vi "JSON File Parse String.vi"(8 "error in (no error)":errorcluster, 11 "file json string":string) -> (0 "error out":errorcluster, 1 "version substring":string, 2 "dsf version substring":string, 3 "dsf configuration substring":string)   [LabVIEW 2017, in "DSF Core.lvlib" / "Configuration Session.lvclass"]
uses:
  Configuration Session.lvclass
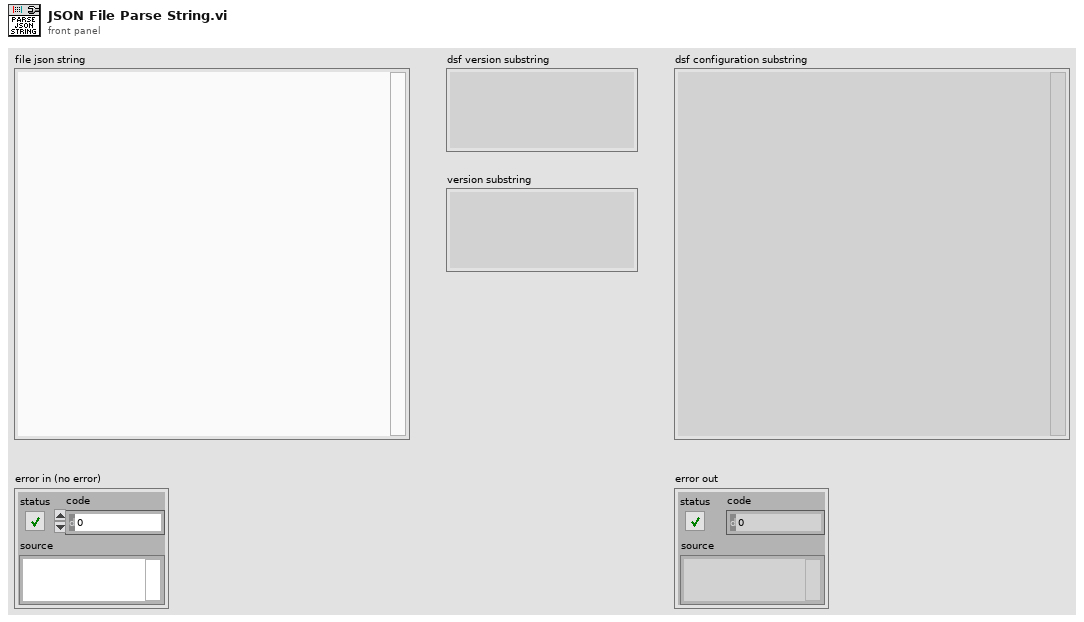
[diagram p1: front panel]
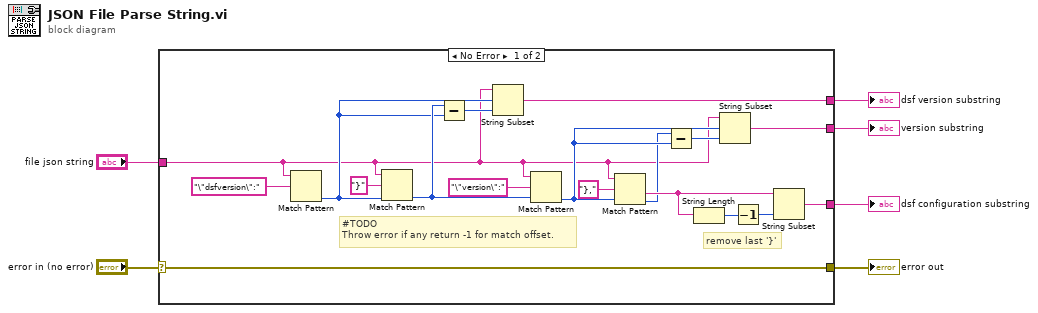
[diagram p0: block diagram]
diagram:
  n1 = case shown="No Error" "error in (no error)" {
    selector: "error in (no error)" -> [w10 w25]
    tunnel: [w19 _] -> w6
    tunnel: "file json string" -> [w7 _]
    tunnel: [w13 _] -> w4
    tunnel: [w12 _] -> w3
    tunnel: [w10 w25] -> w1
    frame No Error {
      # "#TODO\nThrow error if any return -1 for match offset."
      # "remove last '}'"
      n2 = Match Pattern(string=w7, regular expression="\"dsfversion\":") -> (offset past match=w15:i32)  [unwired: 1 in, 3 out]
      n3 = Match Pattern(string=w7, regular expression="}", offset (0)=w15) -> (offset past match=w16:i32)  [unwired: 3 out]
      n4 = Subtract(x=w16, y=w15) -> (x-y=w14:i32)
      n5 = String Subset(string=w7, offset (0)=w15, length (rest)=w14) -> (substring=w13:string)
      n6 = Match Pattern(string=w7, regular expression="\"version\":", offset (0)=w16) -> (offset past match=w17:i32)  [unwired: 3 out]
      n7 = Match Pattern(string=w7, regular expression="},", offset (0)=w17) -> (after substring=w9:string, offset past match=w8:i32)  [unwired: 2 out]
      n8 = Subtract(x=w8, y=w17) -> (x-y=w18:i32)
      n9 = String Length(string=w9) -> (length=w21:i32)
      n10 = String Subset(string=w7, offset (0)=w17, length (rest)=w18) -> (substring=w12:string)
      n11 = Decrement(x=w21) -> (x-1=w20:i32)
      n12 = String Subset(string=w9, length (rest)=w20) -> (substring=w19:string)  [unwired: 1 in]
    }
    frame Error {
    }
  }
  "dsf version substring" <- w4
  "dsf configuration substring" <- w6
  "version substring" <- w3
  "error out" <- w1
